vi "MUX pair error.vi"(8 "error in (no error)":errorcluster, 9 "channel 2":string, 10 "channel 1":string, 11 "SLSC Switch in":refnum<class "SLSC Switch.lvclass">) -> (0 "error out":errorcluster)   [LabVIEW 2015, in "SLSC Switch.lvlib" / "SLSC Switch.lvclass"]
uses:
  SLSC Switch.lvclass
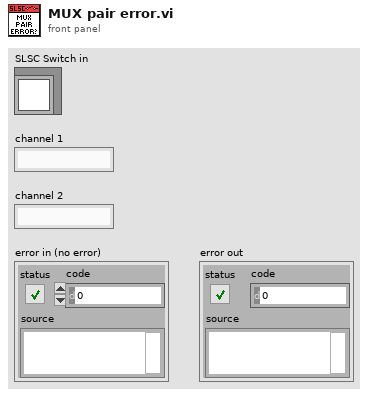
[diagram p1: front panel]
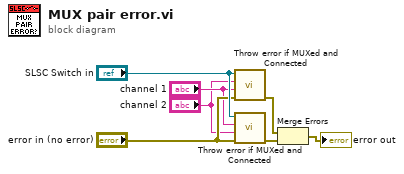
[diagram p0: block diagram]
diagram:
  n1 = call "Throw error if MUXed and Connected.vi"("error in (no error)"="error in (no error)", "Destination"="channel 1", "Source"="channel 2", "SLSC Switch in"="SLSC Switch in") -> ("error out"=w5:errorcluster)  [unwired: 6 in, 1 out]
  n2 = call "Throw error if MUXed and Connected.vi"("error in (no error)"="error in (no error)", "Destination"="channel 2", "Source"="channel 1", "SLSC Switch in"="SLSC Switch in") -> ("error out"=w6:errorcluster)  [unwired: 6 in, 1 out]
  n3 = Merge Errors(w5, w6) -> (→"error out":errorcluster)
